vi "4155C Config Sampling Measurements FPP v2.0.vi"(0 "VISA session":refnum<visa-resource-name>, 1 "Gate Compliance":dbl format="%.2f", 2 "FPP - Source":u32(ring) items=["VSU1  ", "VSU2  "], 3 "FPP - Drain":u32(ring)=1 items=["SMU1  ", "SMU2  ", "SMU3  ", "SMU4  ", "SMU5  ", "SMU6  "], 4 "Drain Compliance":dbl format="%.2f", 5 "error in (no error)":errorcluster, 6 "Num Points":i16=1 min=1 max=1001, 7 "Timings":T2={"integration time"=0, "Short/Long integration time"=0.00064, "hold time (sec)"=0.0, "delay time (sec)"=0.0, "Step Time (0 disables)"=0.0, "sweep method"=0, "Pulse period"=0.005, "Base voltage"=0.0, "Pulse width"=0.0005} {"Pulse width" min=0.0005 max=0.1 step=0.0001 format="%.4f"; "Base voltage" min=-100.0 max=100.0 format="%^.4e"; "Pulse period" min=0.005 max=1.0 step=0.0001 format="%.4f"; "sweep method" items=["Continuous", "Pulsed"]; "Step Time (0 disables)" format="%.2f"; "delay time (sec)" min=0.0 format="%.4f"; "hold time (sec)" min=0.0 format="%.4f"; "Short/Long integration time" min=0.0 format="%^.0e"; "integration time" scale=0.0..2.0}, 8 "FPP - Gate":u32(ring)=2 items=["SMU1  ", "SMU2  ", "SMU3  ", "SMU4  ", "SMU5  ", "SMU6  "], 9 "FPP - Probe 1":u32(ring) items=["SMU1  ", "SMU2  ", "SMU3  ", "SMU4  ", "SMU5  ", "SMU6  "], 10 "Vg":dbl min=-100.0 max=100.0 format="%.2f", 11 "Vd":dbl min=-100.0 max=100.0 format="%.2f", 12 "Display on/off":bool, 13 "Sample time":dbl min=0.0 max=100000000000.0 format="%.2f", 15 "Sampling mode":u32(slide) scale=0.0..4.0, 16 "FPP - Probe 2":u32(ring)=3 items=["SMU1  ", "SMU2  ", "SMU3  ", "SMU4  ", "SMU5  ", "SMU6  "], 18 "Standby":T1) -> (14 "dup VISA resource name":refnum<visa-resource-name>, 19 "error out":errorcluster)   [LabVIEW 2016]
doc: "This VI configures the primary sweep source (VAR1) for a sweep mode measurement. \n* This VI does not perform error checking on MEASUREMENT MODE or UNIT TYPE of VAR1, therefore it is the application programmer's responsibility to make certain this VI is used in the proper mode."
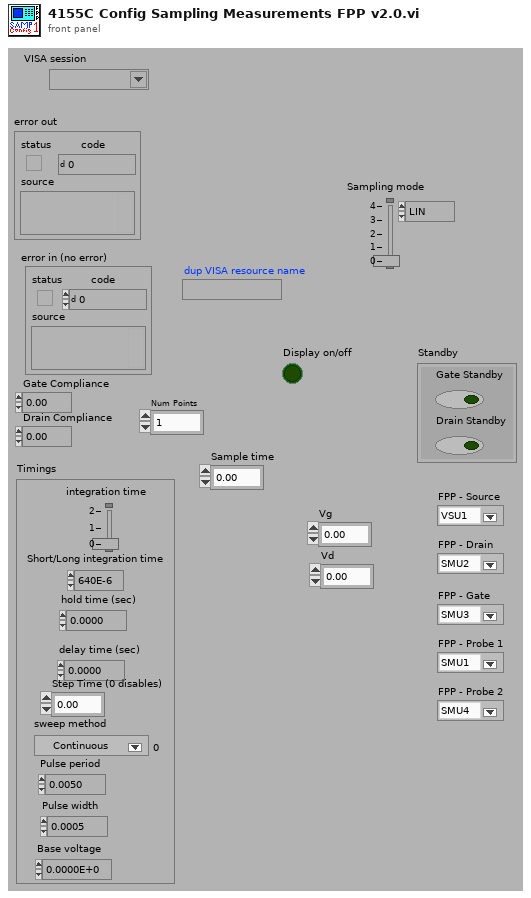
[diagram p1: front panel]
types:
  T1 = cluster{"Gate Standby":bool, "Drain Standby":bool}
  T2 = cluster{"integration time":u32, "Short/Long integration time":dbl, "hold time (sec)":dbl, "delay time (sec)":dbl, "Step Time (0 disables)":dbl, "sweep method":u16, "Pulse period":dbl, "Base voltage":dbl, "Pulse width":dbl}
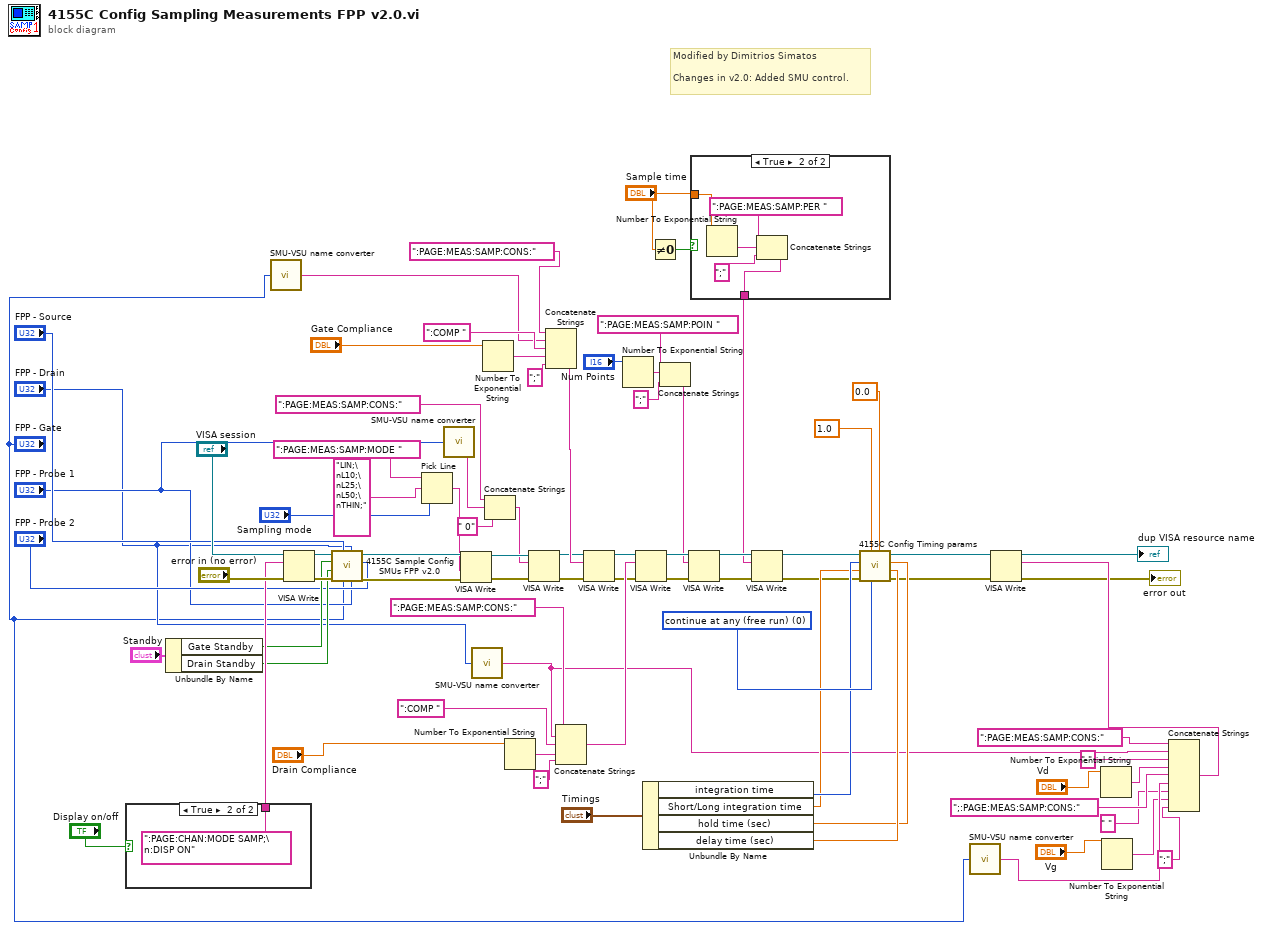
[diagram p0: block diagram]
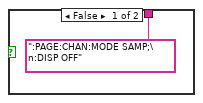
[diagram p2: hidden frame]
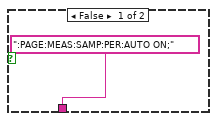
[diagram p3: hidden frame]
diagram:
  w67 = u8 0 items=["continue at any (free run)", "stop at any abnorm", "stop at compliance"] ("stop condition (free run:0)")
  # "Modified by Dimitrios Simatos\n\nChanges in v2.0: Added SMU control."
  n1 = case shown="True" "Display on/off" {
    tunnel: [":PAGE:CHAN:MODE SAMP;\n:DISP OFF" ("write buffer (\"\")") ":PAGE:CHAN:MODE SAMP;\n:DISP ON" ("write buffer (\"\")")] -> w40
    frame False {
    }
    frame True {
    }
  }
  n2 = Unbundle By Name("Standby") -> ("Gate Standby"=w30:bool, "Drain Standby"=w29:bool)
  n3 = call "SMU-VSU name converter.vi"("unit to configure"="FPP - Gate") -> ("SMU/VSU to be configured"=w16:string)
  n4 = VISA Write(VISA resource name="VISA session", write buffer=w40, error in (no error)="error in (no error)") -> (VISA resource name out=w58:refnum<visa-resource-name>, error out=w57:errorcluster)  [unwired: 1 out]
  n5 = call "4155C Sample Config SMUs FPP v2.0.vi"("FPP - Probe 2"="FPP - Probe 2", "FPP - Probe 1"="FPP - Probe 1", "FPP - Drain"="FPP - Drain", "FPP - Gate"="FPP - Gate", "FPP - Source"="FPP - Source", "error in (no error)"=w57, "Drain Standby"=w29, "Gate Standby"=w30, "VISA resource name in"=w58) -> ("error out"=w37:errorcluster, "VISA Resource Name out"=w36:refnum<visa-resource-name>)  [unwired: 1 in]
  n6 = Pick Line(string ("")=":PAGE:MEAS:SAMP:MODE ", multi-line string="LIN;\nL10;\nL25;\nL50;\nTHIN;", line index="Sampling mode") -> (output string=w32:string)
  n7 = call "SMU-VSU name converter.vi"("unit to configure"="FPP - Probe 1") -> ("SMU/VSU to be configured"=w12:string)
  n8 = VISA Write(VISA resource name=w36, write buffer=w32, error in (no error)=w37) -> (VISA resource name out=w39:refnum<visa-resource-name>, error out=w38:errorcluster)  [unwired: 1 out]
  n9 = call "SMU-VSU name converter.vi"("unit to configure"="FPP - Drain") -> ("SMU/VSU to be configured"=w5:string)
  n10 = Number To Exponential String(number="Gate Compliance") -> (E-format string=w74:string)  [unwired: 3 in]
  n11 = Concatenate Strings(":PAGE:MEAS:SAMP:CONS:" ("write buffer (\"\")"), w12, " 0" ("write buffer (\"\")")) -> (w15:string)
  n12 = Number To Exponential String(number="Drain Compliance") -> (E-format string=w76:string)  [unwired: 3 in]
  n13 = VISA Write(VISA resource name=w39, write buffer=w15, error in (no error)=w38) -> (VISA resource name out=w72:refnum<visa-resource-name>, error out=w71:errorcluster)  [unwired: 1 out]
  n14 = Concatenate Strings(":PAGE:MEAS:SAMP:CONS:", w16, ":COMP ", w74, ";" ("Substring")) -> (w75:string)
  n15 = Concatenate Strings(":PAGE:MEAS:SAMP:CONS:", w5, ":COMP ", w76, ";" ("Substring")) -> (w79:string)
  n16 = VISA Write(VISA resource name=w72, write buffer=w75, error in (no error)=w71) -> (VISA resource name out=w70:refnum<visa-resource-name>, error out=w69:errorcluster)  [unwired: 1 out]
  n17 = Number To Exponential String(number="Num Points") -> (E-format string=w55:string)  [unwired: 3 in]
  n18 = VISA Write(VISA resource name=w70, write buffer=w79, error in (no error)=w69) -> (VISA resource name out=w80:refnum<visa-resource-name>, error out=w81:errorcluster)  [unwired: 1 out]
  n19 = Unbundle By Name("Timings") -> ("integration time"=w64:u32, "Short/Long integration time"=w61:dbl, "hold time (sec)"=w65:dbl, "delay time (sec)"=w66:dbl)
  n20 = Not Equal To 0?(x="Sample time") -> (x != 0?=w47:bool)
  n21 = Concatenate Strings(":PAGE:MEAS:SAMP:POIN " ("write buffer (\"\")"), w55, ";" ("Substring")) -> (w49:string)
  n22 = VISA Write(VISA resource name=w80, write buffer=w49, error in (no error)=w81) -> (VISA resource name out=w46:refnum<visa-resource-name>, error out=w45:errorcluster)  [unwired: 1 out]
  n23 = case shown="True" w47 {
    tunnel: "Sample time" -> [_ w88]
    tunnel: [":PAGE:MEAS:SAMP:PER:AUTO ON;" w85] -> w42
    frame False {
    }
    frame True {
      n24 = Number To Exponential String(number=w88) -> (E-format string=w89:string)  [unwired: 3 in]
      n25 = Concatenate Strings(":PAGE:MEAS:SAMP:PER " ("Substring"), w89, ";" ("Substring")) -> (w85:string)
    }
  }
  n26 = VISA Write(VISA resource name=w46, write buffer=w42, error in (no error)=w45) -> (VISA resource name out=w43:refnum<visa-resource-name>, error out=w44:errorcluster)  [unwired: 1 out]
  n27 = call "4155C Config Timing params.vi"("delay time (sec)"=w66, "hold time (sec)"=w65, "Step Time (0 disables)"=0.0, "stop condition (free run:0)"=w67, "wait time parameter"=1.0, "error in (no error)"=w44, "Short/Long integration time"=w61, "integration time"=w64, "VISA session"=w43) -> ("error out"=w22:errorcluster, "dup VISA resource name"=w23:refnum<visa-resource-name>)  [unwired: 1 in]
  n28 = call "SMU-VSU name converter.vi"("unit to configure"="FPP - Gate") -> ("SMU/VSU to be configured"=w8:string)
  n29 = Number To Exponential String(number="Vd") -> (E-format string=w27:string)  [unwired: 3 in]
  n30 = Number To Exponential String(number="Vg") -> (E-format string=w2:string)  [unwired: 3 in]
  n31 = Concatenate Strings(":PAGE:MEAS:SAMP:CONS:" ("write buffer (\"\")"), w5, " " ("string"), w27, ";:PAGE:MEAS:SAMP:CONS:" ("write buffer (\"\")"), w8, " " ("string"), w2, ";" ("Substring")) -> (w24:string)
  n32 = VISA Write(VISA resource name=w23, write buffer=w24, error in (no error)=w22) -> (VISA resource name out=→"dup VISA resource name":refnum<visa-resource-name>, error out=→"error out":errorcluster)  [unwired: 1 out]
